vi "Stop Core.vi"(10 "最终错误代码":i32, 11 "客户端输入":refnum<class "客户端.lvclass">) -> (3 "客户端输出":refnum<class "客户端.lvclass">)   [LabVIEW 2015, in "客户端操作者.lvlib" / "客户端.lvclass"]
doc: "对于操作者运行过程中创建的所有并行进程，在重写Stop Core.vi的VI中应调用必要代码使其停止运行。需要停止的进程包括该操作本身创建的层层嵌套的操作者，以及所有其他异步运行的VI，比如时间延迟消息。需要停止的进程可能还包括Actor Core中的所有并行循环。（另一种方法，是在Actor Core程序框图上，在“调用父节点”结束时触发一个局部信号来停止这些进程。）\n\n<b>最终错误代码</b>输入表示操作者退出时设定的错误。0表示无错误。该错误代码可用于区分“正常停止”和“紧急停止”，从而向其他操作者发送信号。一般用非零值表示“紧急停止”，当然对于某个特定的操作者也可采用其他的表示方法。请注意，1608是个特殊的错误代码，表示当前操作者本身被“紧急停止”，如出现该错误，只能直接传递该代码。"
uses:
  <vilib>/ActorFramework/Actor/Actor.lvclass
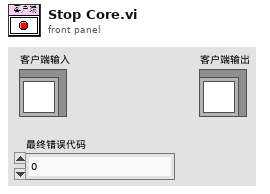
[diagram p1: front panel]
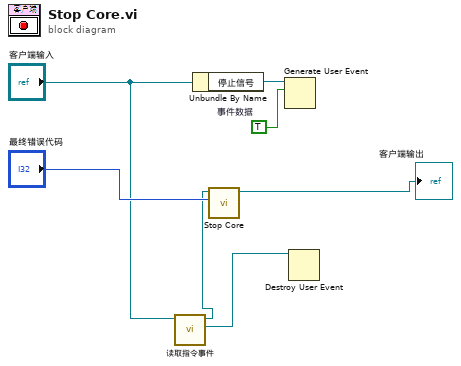
[diagram p0: block diagram]
diagram:
  w5 = TRUE  # 事件数据
  n1 = call-dynamic "读取指令事件.vi"("客户端输入"="客户端输入") -> ("指令事件"=w4:refnum<user-event>, "客户端输出"=w1:refnum<class "客户端.lvclass">)  [unwired: 8 in, 1 out]
  n2 = Unbundle By Name("客户端输入") -> ("停止信号"=w6:refnum<user-event>)
  n3 = call-parent "Stop Core.vi"("final error code"="最终错误代码", "Actor in"=w1) -> ("Actor out"=→"客户端输出":refnum<class "客户端.lvclass">)  [unwired: 9 in]
  n4 = Generate User Event(user event=w6, event data cluster=w5) -> ()  [unwired: 2 in, 2 out]
  n5 = Destroy User Event(user event=w4) -> ()  [unwired: 1 in, 1 out]
